vi "Граница.vi"(0 "Перерасчет":dbl[](array[numeric]), 1 "Time":dbl[](array[numeric]), 2 "Atm":dbl[](array[numeric]), 3 "Вип":dbl[](array[numeric]), 4 "Граница":dbl) -> (5 "time":dbl, 6 "Вип":dbl, 7 "Atm":dbl, 8 "Numeric 4":i32)   [LabVIEW 2018]
panel:
  out "Первый":bool
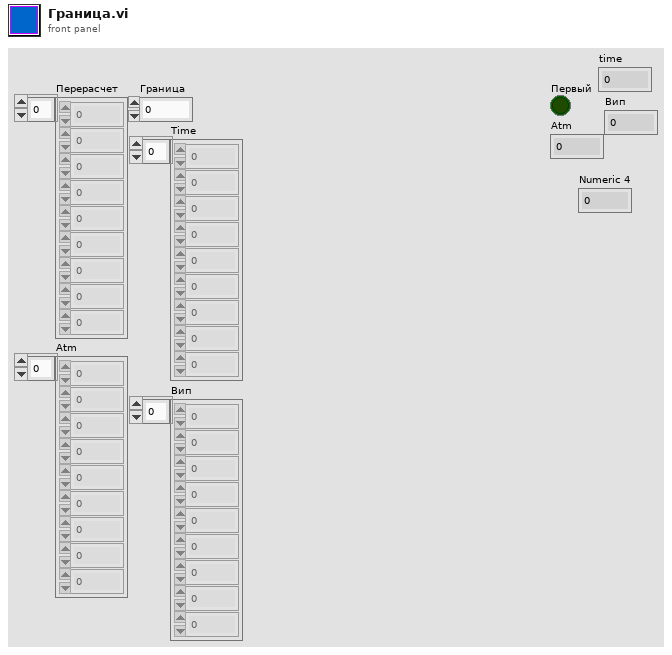
[diagram p1: front panel]
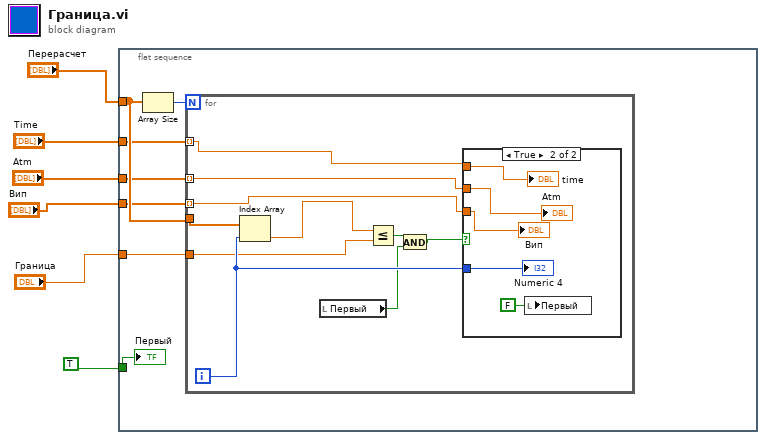
[diagram p0: block diagram]
diagram:
  n1 = flat-sequence {
    tunnel: TRUE ("Первый") -> [w10]
    tunnel: "Граница" -> [w12]
    tunnel: "Перерасчет" -> [w11]
    tunnel: "Time" -> [w9]
    tunnel: "Atm" -> [w8]
    tunnel: "Вип" -> [w7]
    frame #0 {
      n2 = Array Size(array=w11) -> (size(s)=w13:i32)
      n3 = for {
        N: w13 -> [_]
        tunnel: w11 -> [w23]
        tunnel: w12 -> [w21]
        tunnel: w9 -> [w16] mode=indexing
        tunnel: w8 -> [w15] mode=indexing
        tunnel: w7 -> [w14] mode=indexing
        i -> [w22]
        n4 = Index Array(array=w23, index=w22) -> (element=w20:dbl)
        n5 = local read "Первый"() -> (w17:bool)
        n6 = Less Or Equal?(x=w20, y=w21) -> (x <= y?=w19:bool)
        n7 = And(x=w19, y=w17) -> (x .and. y?=w18:bool)
        n8 = case shown="True" w18 {
          tunnel: w22 -> [_ w28]
          tunnel: w16 -> [_ w26]
          tunnel: w15 -> [_ w25]
          tunnel: w14 -> [_ w24]
          frame False {
          }
          frame True {
            n9 = local write "Первый"(FALSE ("Первый")) -> ()
            "Numeric 4" <- w28
            "time" <- w26
            "Atm" <- w25
            "Вип" <- w24
          }
        }
      }
      "Первый" <- w10
    }
  }
